vi "Game Controller Teleop.vi"(10 "Match Info":T13={"Autonomous Elapsed Seconds"=0.0, "TeleOp Elapsed Seconds"=0.0, "Disabled Elapsed Seconds"=0.0, "Visited Autonomous"=FALSE, "Visited TeleOp"=FALSE, "Visited Disabled"=FALSE, "Autonomous Settings"={"Autonomous Style"=enum."Independent", "VI Refnum"=refnum}}, 11 "Call Context":T14) -> ()   [LabVIEW 2020]
doc: "This VI is called for each TeleOp packet received from the DS where the robot is not disabled. It is often used to read from the joysticks and update I/O or to update setpoints for timed control loops. It should complete and return within 20 milliseconds or it may miss DS packets."
uses:
  <vilib>/Rock Robotics/WPI/DriverStation/WPI_DriverStationDerivedRobotMode.ctl
  <vilib>/Rock Robotics/WPI/DriverStation/WPI_DriverStationMatch Info.ctl
  Shared Code/TypeDefs/Cluster_Extend HW Outputs.ctl
  Shared Code/TypeDefs/Cluster_FX CloseLoop Values.ctl
  Shared Code/TypeDefs/Cluster_FX Limit Switchs.ctl
  Shared Code/TypeDefs/Cluster_FX Current Values.ctl
  Shared Code/TypeDefs/Cluster_FX Sensor Values.ctl
  Shared Code/TypeDefs/Cluster_FX Integrated Sensor Values.ctl
  Shared Code/TypeDefs/Cluster_Sholder_HW Outputs.ctl
  Shared Code/TypeDefs/Cluster_Wrist HW Outputs.ctl
  Shared Code/TypeDefs/Cluster_Pose Positions.ctl
  Systems/MotionMaser/ENUM_Pose List.ctl
  Type Defs/Cluster_Pigeon Tilt Data.ctl
  Shared Code/TypeDefs/ENUM_Tilt State.ctl
  Systems/SwerveDrive/Cluster_CMD_ACT_Data.ctl
  Shared Code/TypeDefs/ENUM_Swerve_CMD_Mode Select.ctl
  Shared Code/TypeDefs/Cluster_CMD_Direction Data.ctl
  Shared Code/TypeDefs/Cluster_Module Velocity-Direction-Rotations.ctl
  Shared Code/TypeDefs/Level_Velocity plus-minus 1.ctl
  Shared Code/TypeDefs/Dial_Compase heading unit circle CCW positive.ctl
  Type Defs/NUM_Rotate Input.ctl
  Shared Code/TypeDefs/Cluster_X-Y.ctl
  Systems/PigeonIMU/Cluster_CMD_SEN_Data.ctl
  Teleop Support/ENUM_Button Select.ctl
  Teleop Support/ENUM_Axes Select.ctl
  Systems/Extention/Cluster_CMD_ACT_Data.ctl
  Shared Code/TypeDefs/ENUM_Extend_CMD_Mode Select.ctl
  Systems/Sholder/Cluster_CMD_ACT_Data.ctl
  Shared Code/TypeDefs/ENUM_Sholder_CMD_Mode Select.ctl
  Systems/Wrist/Cluster_CMD_ACT_Data.ctl
  Shared Code/TypeDefs/ENUM_Wrist_CMD_Mode Select.ctl
  Systems/Grabber/Cluster_CMD_ACT_Data.ctl
  Shared Code/TypeDefs/ENUM_Grabber_CMD_Mode Select.ctl
  Shared Code/TypeDefs/ENUM_Controller Buzz Select.ctl
  3c76d165-6d6f-4521-944b-83df467126d5.vi
  5b221245-1683-49e4-bbda-b419f5af282c.vi
  8735cd3c-726f-4517-be5d-f0f5cfaf1625.vi
  <vilib>/Rock Robotics/Network Tables/NT Write Boolean.vi
  Systems/Game Controller/Global_SEN_Data Out.vi
  Systems/PigeonIMU/Global_CMD_SEN_Data In.vi
  Systems/Grabber/Global_CMD_ACT_Data In.vi
  Systems/Wrist/Global_CMD_ACT_Data In.vi
  Systems/Extention/Global_ACT_Data Out.vi
  Systems/Sholder/Global_ACT_Data Out.vi
  Systems/Wrist/Global_ACT_Data Out.vi
  Systems/Extention/Global_CMD_ACT_Data In.vi
  Systems/Grabber/Global_ACT_Data Out.vi
  Systems/Game Controller/Global_CMD_Data In.vi
  Systems/SwerveDrive/Global_CMD_ACT_Data In.vi
  Systems/Sholder/Global_CMD_ACT_Data In.vi
  Systems/PigeonIMU/Global_SEN_Data Out.vi
  Systems/SwerveDrive/Global_ACT_Data Out.vi
  <vilib>/Comparison/Equal/Equal Functor/Equal Functor.lvclass
  Systems/Game Controller/GameController_SEN.lvlib
  Systems/SwerveDrive/SwerveDrive_ACT.lvlib
  Systems/PigeonIMU/PigeonIMU_SEN.lvlib
  Systems/Extention/Extend_ACT.lvlib
  Systems/Sholder/Sholder_ACT.lvlib
  Systems/Wrist/Wrist_ACT.lvlib
  Systems/Grabber/Grabber_ACT.lvlib
  Systems/MotionMaser/MotionMaster_SubCMD.lvlib
panel:
  out "Rotation Reduction":dbl
  in  "Balance speed (ft/s)":dbl=10.0
  out "Sen_Pigeon_Tilt Data":T1
  out "Pose":T3
  out "Target  Position Out":T4
  in  "Min Translation Speed (ft/s)":dbl=2.0 format="%#_13g"
  in  "max rotation speed":dbl=0.4
  in  "shoulder speed":dbl=-0.3
  out "ACT_Wrist_HW Output":T5
  out "ACT_Sholder_HW Outputs":T11
  out "ACT_Extend_HW Outputs":T12
  out "POSITION":bool
  in  "funny tilt button":bool
  in  "Drive Deadband":dbl=0.25 format="%#_13g"
  in  "Rotation Deadband":dbl=0.15 format="%#_13g"
  in  "Square Throttle?":bool
  in  "Square Joystick Inputs?":bool
  in  "Max Translation Speed (ft/s)":dbl=16.0 format="%#_13g"
  out "POV":i16
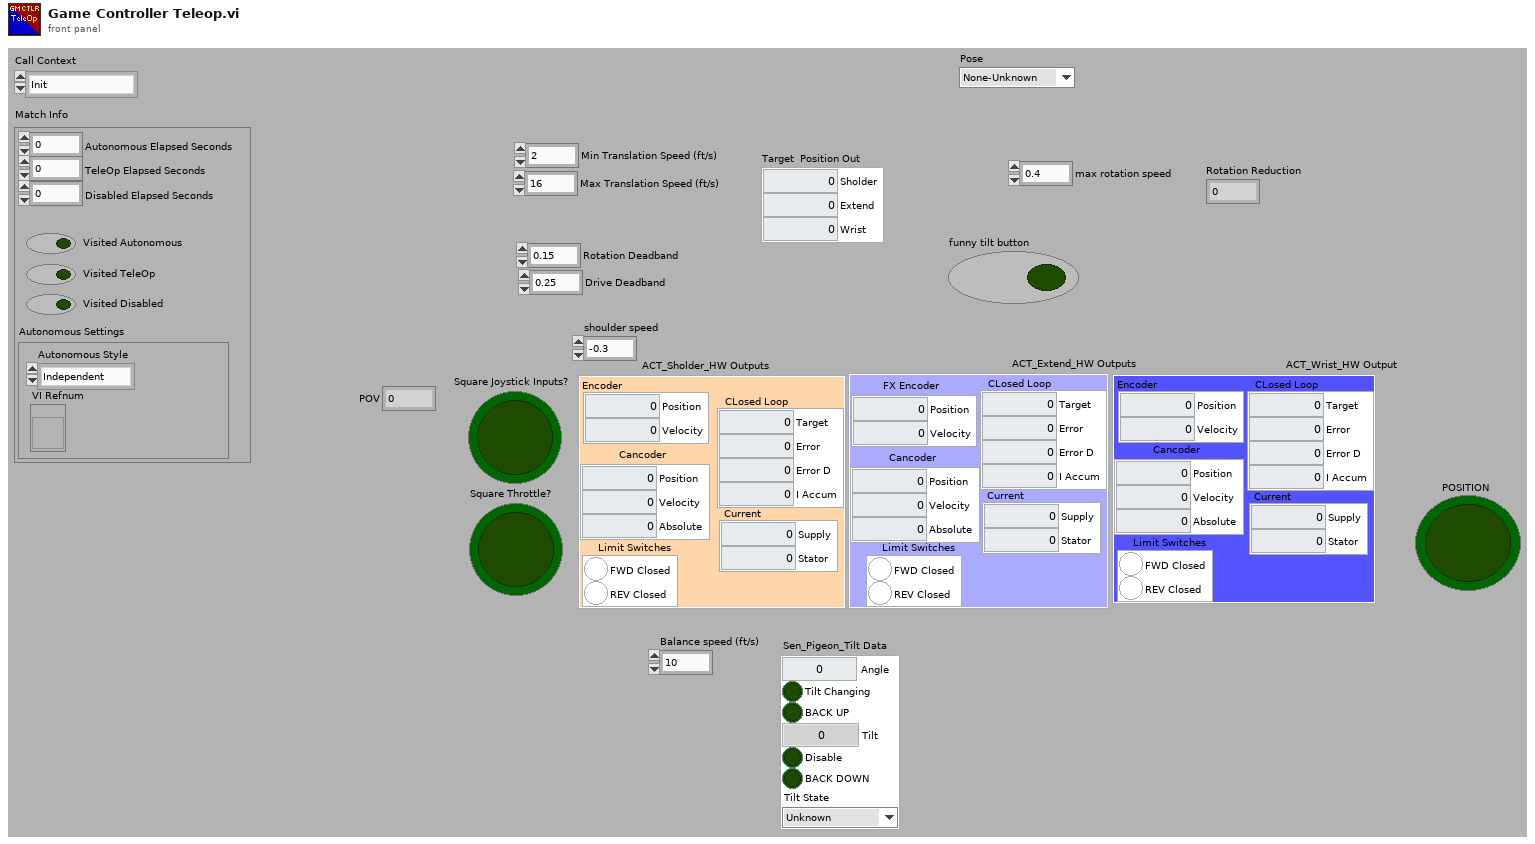
[diagram p1: front panel]
types:
  T1 = typedef "Cluster_Pigeon Tilt Data.ctl" = cluster{"Angle":dbl, "Tilt Changing":bool, "BACK UP":bool, "Tilt":dbl, "Disable":bool, "BACK DOWN":bool, "Tilt State":T2}
  T2 = typedef "ENUM_Tilt State.ctl" = enum16{"Unknown", "Level", "Angle UP from Level", "Level from Angle Up", "Angle Down from Level", "Level from Angle Down"}
  T3 = typedef "MotionMaster_SubCMD.lvlib/ENUM_Pose List.ctl" = enum16{"None-Unknown", "Intake", "Score High", "Score Mid", "Safe Position", "Home Pos"}
  T4 = typedef "Cluster_Pose Positions.ctl" = cluster{"Sholder":i32, "Extend":i32, "Wrist":i32}
  T5 = typedef "Cluster_Wrist HW Outputs.ctl" = cluster{"Encoder":T6, "CLosed Loop":T7, "Limit Switches":T8, "Current":T9, "Cancoder":T10}
  T6 = typedef "Cluster_FX Sensor Values.ctl" = cluster{"Position":i32, "Velocity":i32}
  T7 = typedef "Cluster_FX CloseLoop Values.ctl" = cluster{"Target":dbl, "Error":i32, "Error D":dbl, "I Accum":dbl}
  T8 = typedef "Cluster_FX Limit Switchs.ctl" = cluster{"FWD Closed":bool, "REV Closed":bool}
  T9 = typedef "Cluster_FX Current Values.ctl" = cluster{"Supply":dbl, "Stator":dbl}
  T10 = typedef "Cluster_FX Integrated Sensor Values.ctl" = cluster{"Position":dbl, "Velocity":dbl, "Absolute":dbl}
  T11 = typedef "Cluster_Sholder_HW Outputs.ctl" = cluster{"Encoder":T6, "CLosed Loop":T7, "Limit Switches":T8, "Current":T9, "Cancoder":T10}
  T12 = typedef "Cluster_Extend HW Outputs.ctl" = cluster{"CLosed Loop":T7, "Limit Switches":T8, "Current":T9, "FX Encoder":T6, "Cancoder":T10}
  T13 = typedef "WPI_DriverStationMatch Info.ctl" = cluster{"Autonomous Elapsed Seconds":dbl, "TeleOp Elapsed Seconds":dbl, "Disabled Elapsed Seconds":dbl, "Visited Autonomous":bool, "Visited TeleOp":bool, "Visited Disabled":bool, "Autonomous Settings":cluster{"Autonomous Style":enum16{"Iterative", "Independent"}, "VI Refnum":refnum<vi>}}
  T14 = typedef "WPI_DriverStationDerivedRobotMode.ctl" = enum16{"Init", "Execute", "Stop"}
  T15 = typedef "ENUM_Button Select.ctl" = enum16{"RightPad Green A", "RightPad Red B", "RightPad Blue X", "RightPad Yellow Y", "Left Bump", "Right Bump", "CenterPad Back", "CenterPad Start", "LeftStick Press", "RightStick Press"}
  T16 = typedef "ENUM_Swerve_CMD_Mode Select.ctl" = enum16{"Coast", "Manual", "Auto Trans Auto Rotate", "Manual Trans Auto Rotate", "Balance", "Stop Brake", "Lock Wheels"}
  T17 = typedef "ENUM_Extend_CMD_Mode Select.ctl" = enum16{"STOP", "Position", "Velocity", "Force Home"}
  T18 = typedef "ENUM_Axes Select.ctl" = enum16{"Left Stick Left (-1) Right (1)", "Left Stick Fwd (-1) Back(1)", "Left Trigger (0-1)", "Right Trigger (0-1)", "Right Stick Left(-1 Right (1)", "Right Stick Fwd(-1) Back (1)"}
  T19 = typedef "NUM_Rotate Input.ctl" = dbl
  T20 = typedef "Dial_Compase heading unit circle CCW positive.ctl" = dbl
  T21 = typedef "ENUM_Grabber_CMD_Mode Select.ctl" = enum16{"STOP", "Intake", "Eject"}
  T22 = typedef "Grabber_ACT.lvlib/Cluster_CMD_ACT_Data.ctl" = cluster{"Mode":T21}
  T23 = typedef "Wrist_ACT.lvlib/Cluster_CMD_ACT_Data.ctl" = cluster{"Mode":T24, "Position (counts)":i32, "Velocity (0-1)":dbl}
  T24 = typedef "ENUM_Wrist_CMD_Mode Select.ctl" = enum16{"STOP", "Position", "Speed"}
  T25 = typedef "Sholder_ACT.lvlib/Cluster_CMD_ACT_Data.ctl" = cluster{"Mode":T26, "Position (counts)":i32, "Velocity (0-1)":dbl}
  T26 = typedef "ENUM_Sholder_CMD_Mode Select.ctl" = enum16{"STOP", "Position", "Percent out"}
  T27 = typedef "Extend_ACT.lvlib/Cluster_CMD_ACT_Data.ctl" = cluster{"Mode":T17, "Position (counts)":i32, "Velocity (0-1)":dbl}
  T28 = typedef "PigeonIMU_SEN.lvlib/Cluster_CMD_SEN_Data.ctl" = cluster{"Reset":bool, "Disable":bool}
  T29 = typedef "Cluster_Module Velocity-Direction-Rotations.ctl" = cluster{"Velocity":T30, "Angle":T20, "Rotations Count":dbl}
  T30 = typedef "Level_Velocity plus-minus 1.ctl" = dbl
  T31 = typedef "SwerveDrive_ACT.lvlib/Cluster_CMD_ACT_Data.ctl" = cluster{"Mode":T16, "Direction":T32, "Orientation Robot(t) Field(f)":bool, "Max Translation Speed (ft/sec)":dbl, "Rotation Reduction 1-0":dbl, "Rotation Center From Robot Center":T33, "Auto Angle":T20, "Auto Target (ft)":dbl}
  T32 = typedef "Cluster_CMD_Direction Data.ctl" = cluster{"Traverse":T29, "Rotate(Yaw) CCW 1 CW -1":T19}
  T33 = typedef "Cluster_X-Y.ctl" = cluster{"X":dbl, "Y":dbl}
  T34 = typedef "Cluster_Grabber_SW Outputs.ctl" = cluster{"Enabled":bool, "Closed Loop":bool, "Stalled":bool}
  T35 = typedef "GameController_SEN.lvlib/ENUM_SEN_State.ctl" = enum16{"Startup", "Waiting BUZZ ON", "Shutdown", "Buzzing FULL Timed", "Waiting BUZZ OFF", "Buzzing Cycle Count", "Buzzing Intensity"}
  T36 = typedef "ENUM_Controller Buzz Select.ctl" = enum16{"None", "Timed Full ON", "Set Intensity", ".5 Sec Cycle Count"}
  T37 = typedef "Cluster_Config_Balance Data.ctl" = cluster{"BalancePID Ver":u64, "PID":T38}
  T38 = typedef "Cluster_PID Config.ctl" = cluster{"Gains":T39, "Error Allowed":T40, "I Zone":T40, "Max Out":T41, "Max I Accu":T40, "CL Ramp Rate (S)":dbl}
  T39 = typedef "Cluster_PID Gains.ctl" = cluster{"P":dbl, "I":dbl, "D":dbl, "F":dbl}
  T40 = typedef "Cluster_High-Low.ctl" = cluster{"High":dbl, "Low":dbl}
  T41 = typedef "Cluster_FWD  REV Values.ctl" = cluster{"FWD":dbl, "REV":dbl}
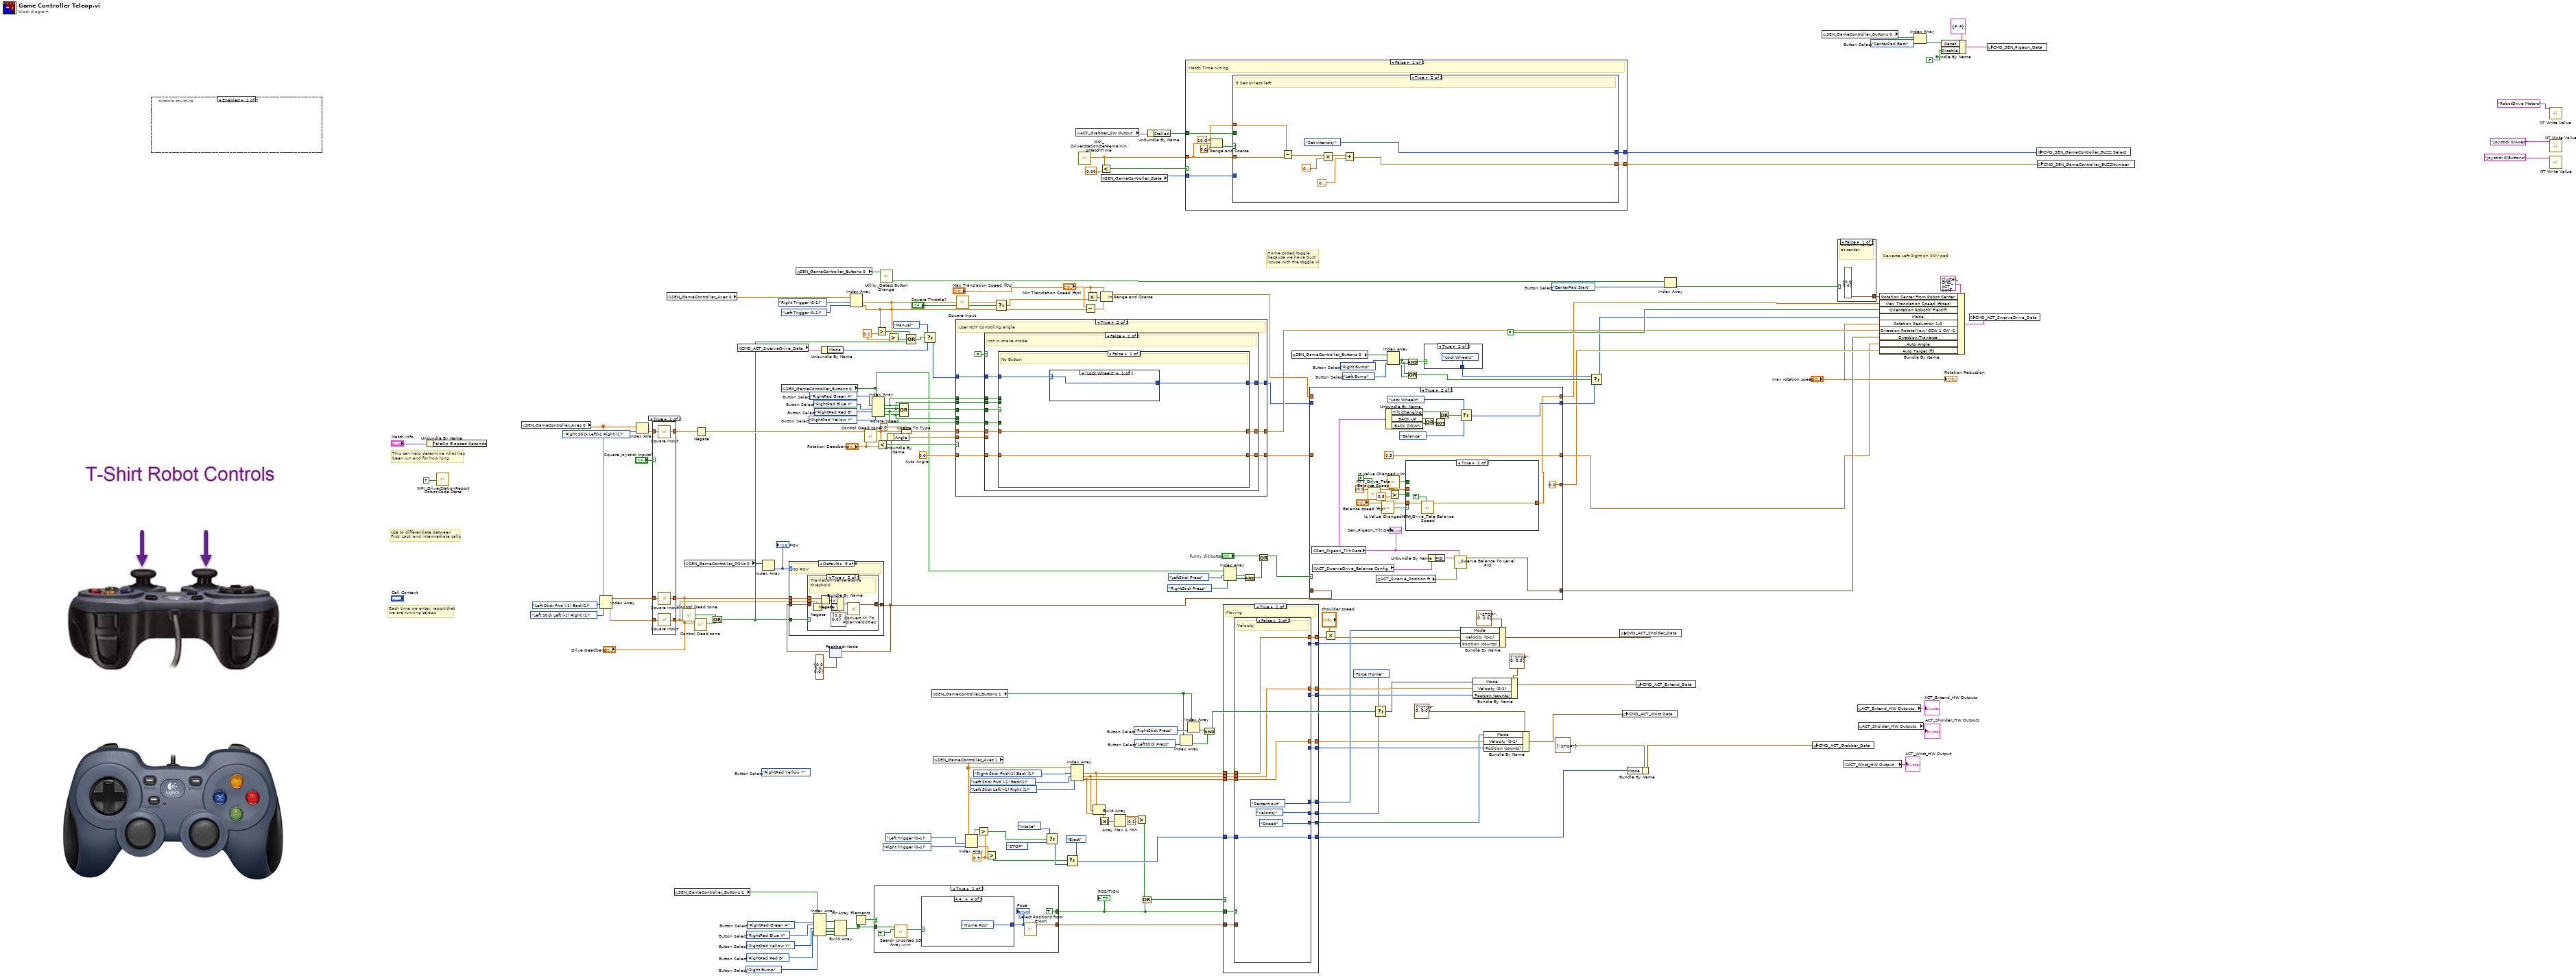
[diagram p0: block diagram]
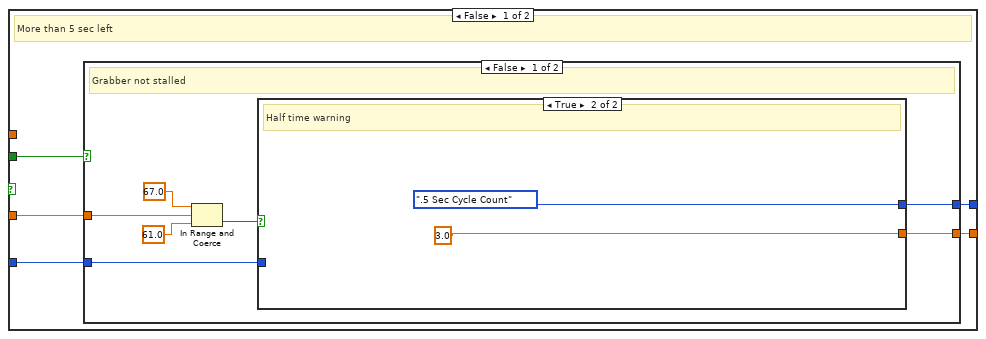
[diagram p2: hidden frame]
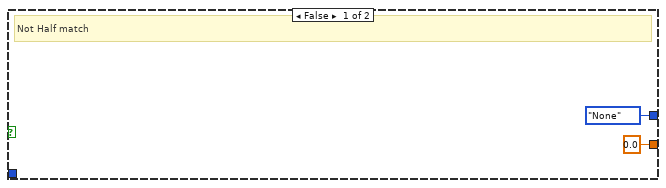
[diagram p3: hidden frame]
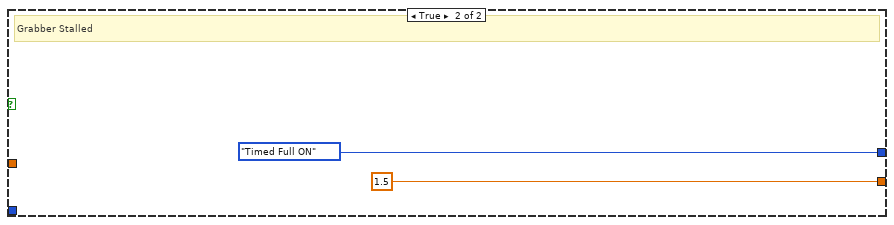
[diagram p4: hidden frame]
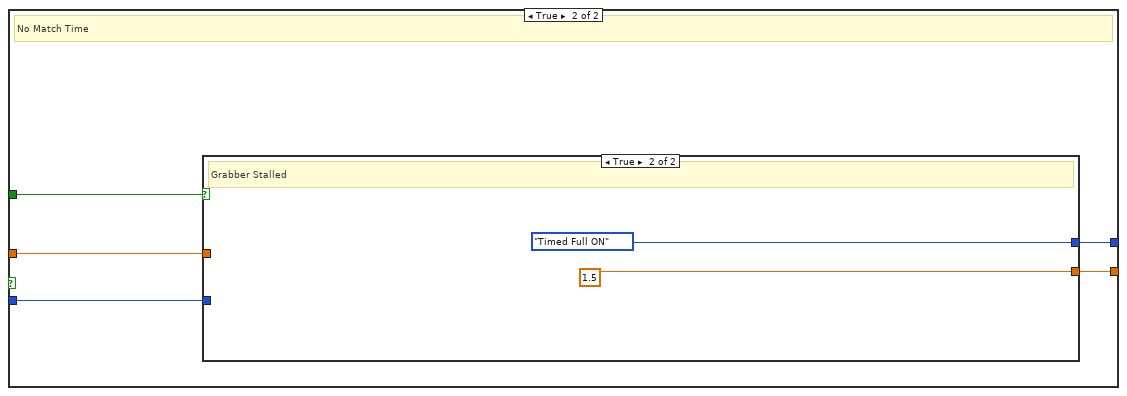
[diagram p5: hidden frame]
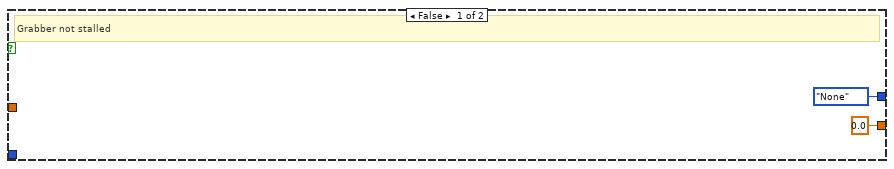
[diagram p6: hidden frame]
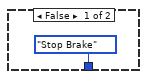
[diagram p7: hidden frame]
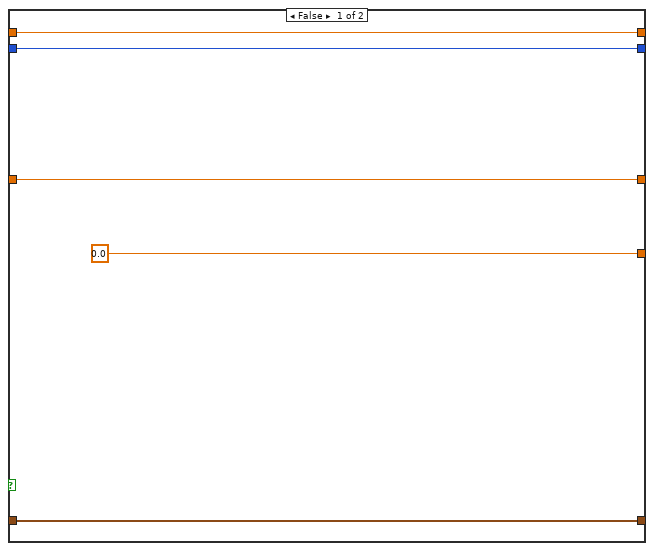
[diagram p8: hidden frame]
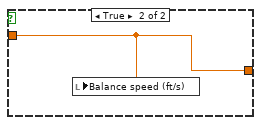
[diagram p11: hidden frame]
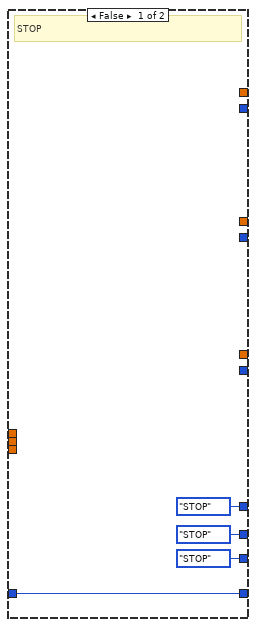
[diagram p12: hidden frame]
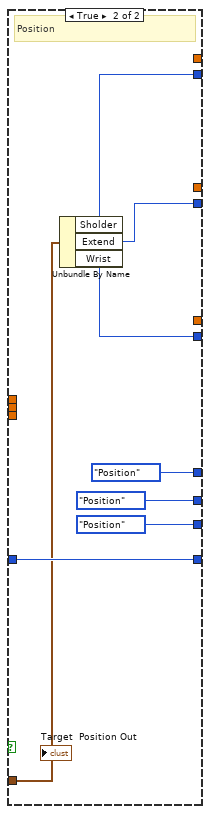
[diagram p13: hidden frame]
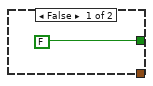
[diagram p14: hidden frame]
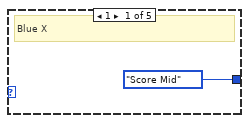
[diagram p15: hidden frame]
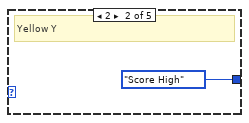
[diagram p16: hidden frame]
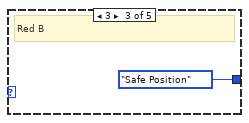
[diagram p17: hidden frame]
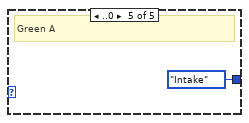
[diagram p18: hidden frame]
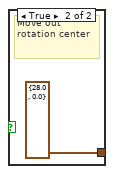
[diagram p19: hidden frame]
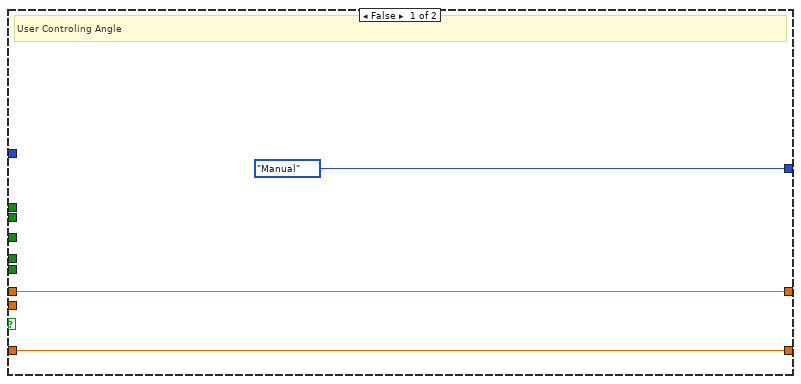
[diagram p20: hidden frame]
diagram:
  w22 = 0.1 ("y")
  w42 = ENUM_Button_Select."Left Bump"  # Button Select
  w51 = ENUM_Button_Select."LeftStick Press"  # Button Select
  w76 = T19 0.0  # Rotate Speed
  w79 = T20 0.0  # Auto Angle
  w82 = ENUM_Button_Select."Right Bump"  # Button Select
  w99 = ENUM_Button_Select."RightPad Red B"  # Button Select
  w100 = ENUM_Button_Select."RightPad Yellow Y"  # Button Select
  w101 = ENUM_Button_Select."RightPad Blue X"  # Button Select
  w102 = ENUM_Button_Select."RightPad Green A"  # Button Select
  (unwired) ENUM_Button_Select."RightPad Yellow Y"  # Button Select
  w109 = 0.9 ("y")
  w145 = ENUM_Button_Select."RightStick Press"  # Button Select
  w155 = ENUM_Button_Select."RightPad Yellow Y"  # Button Select
  w156 = ENUM_Button_Select."RightPad Red B"  # Button Select
  w157 = ENUM_Button_Select."RightPad Blue X"  # Button Select
  w165 = ENUM_Button_Select."CenterPad Start"  # Button Select
  w166 = ENUM_Button_Select."Right Bump"  # Button Select
  w170 = ENUM_Button_Select."CenterPad Back"  # Button Select
  w168 = ENUM_Button_Select."RightPad Green A"  # Button Select
  # "Home coded toggle\nbecause we have trust\nissuse with the toggle VI"
  # "Reverse Left Right on POV pad"
  # "Each time we enter, report that\nwe are running teleop"
  # "Use to differentiate between\nFirst, Last, and Intermediate calls"
  # "This can help determine what has\nbeen run and for how long"
  n1 = disable-structure shown="Enabled" {
    frame Disabled {
      n2 = global read "Global_SEN_Data Out.vi" "SEN_GameController_Axes 1"() -> (w184:dbl[])
      n3 = global read "Global_SEN_Data Out.vi" "SEN_GameController_POVs 1"() -> (w183:i16[])
      n4 = global read "Global_SEN_Data Out.vi" "SEN_GameController_Buttons 1"() -> ()  [unwired: 1 out]
      n5 = Index Array(array=w183) -> ()  [unwired: 1 in, 1 out]
      n6 = Index Array(array=w184) -> ()  [unwired: 1 in, 1 out]
    }
    frame Enabled {
    }
  }
  n7 = Unbundle By Name("Match Info") -> ()  [unwired: 1 out]
  n8 = call <vilib>:"WPI_DriverStationReport Robot Code State.vi"("TeleOp"=TRUE ("Autonomous")) -> ()  [unwired: 10 in, 1 out]
  n9 = global read "Global_SEN_Data Out.vi" "SEN_GameController_Axes 0"() -> (w138:dbl[])
  n10 = Index Array(array=w138, index #1=ENUM_Axes_Select."Left Stick Fwd (-1) Back(1)" ("Axes Select"), index #2=ENUM_Axes_Select."Left Stick Left (-1) Right (1)" ("Axes Select")) -> (element #1=w161:dbl, element #2=w134:dbl)
  n11 = Index Array(array=w138, index=ENUM_Axes_Select."Right Stick Left(-1 Right (1)" ("Axes Select")) -> (element=w136:dbl)
  n12 = case shown="True" "Square Joystick Inputs?" {
    tunnel: [w185 w188] -> w162
    tunnel: [w186 w189] -> w1
    tunnel: [w187 w190] -> w2
    tunnel: w161 -> [w187 w193]
    tunnel: w136 -> [w185 w191]
    tunnel: w134 -> [w186 w192]
    frame False {
    }
    frame True {
      n13 = call "Square Input.vi"("Input"=w191) -> ("Output Squared"=w188:dbl)
      n14 = call "Square Input.vi"("Input"=w193) -> ("Output Squared"=w190:dbl)
      n15 = call "Square Input.vi"("Input"=w192) -> ("Output Squared"=w189:dbl)
    }
  }
  n16 = global read "Global_SEN_Data Out.vi" "SEN_GameController_Axes 0"() -> (w141:dbl[])
  n17 = global read "Global_SEN_Data Out.vi" "SEN_GameController_Buttons 1"() -> (w84:bool[])
  n18 = call "Control Dead zone.vi"("dead zone"="Drive Deadband", "control Value"=w2) -> ("Active"=w69:bool)  [unwired: 8 in, 1 out]
  n19 = global read "Global_SEN_Data Out.vi" "SEN_GameController_POVs 0"() -> (w177:i16[])
  n20 = call "Control Dead zone.vi"("dead zone"="Drive Deadband", "control Value"=w1) -> ("Active"=w70:bool)  [unwired: 8 in, 1 out]
  n21 = Negate(x=w162) -> (-x=w73:dbl)
  n22 = Or(x=w69, y=w70) -> (x .or. y?=w17:bool)
  n23 = global read "Global_CMD_ACT_Data In.vi" "CMD_ACT_SwerveDrive_Data"() -> (w27:T31)
  n24 = Index Array(array=w177) -> (element=w144:i16)  [unwired: 1 in]
  "POV" <- w144
  n25 = global read "Global_SEN_Data Out.vi" "SEN_GameController_Buttons 0"() -> (w16:bool[])
  n26 = global read "Global_SEN_Data Out.vi" "SEN_GameController_Buttons 0"() -> (w53:bool[])
  n27 = Index Array(array=w84, index #1=w102, index #2=w101, index #3=w100, index #4=w99, index #5=w82) -> (element #1=w98:bool, element #2=w97:bool, element #3=w96:bool, element #4=w95:bool, element #5=w81:bool)
  n28 = Unbundle By Name(w27) -> ("Mode"=w20:T16)
  n29 = feedback #1(T29 {"Velocity"=0.0, "Angle"=0.0, "Rotations Count"=0.0} ("Polar Out")) -> (w72:T29)
  n30 = case shown="Default" w144 {
    tunnel: w2 -> [_ _ _ _ _ _ _ _ w230]
    tunnel: w1 -> [_ _ _ _ _ _ _ _ w229]
    tunnel: w72 -> [w197 w201 w205 w209 w213 w217 w221 w225 w228]
    tunnel: [w194 w198 w202 w206 w210 w214 w218 w222 w227] -> w9
    tunnel: w17 -> [_ _ _ _ _ _ _ _ w226]
    frame 0 {
      # "POV Forward"
      n31 = Bundle By Name(cluster=w197, "Velocity"=T30 1.0, "Angle"=T20 0.0) -> (w194:T29)
    }
    frame 45 {
      # "POV Forward Right"
      n32 = Bundle By Name(cluster=w201, "Velocity"=T30 1.0, "Angle"=T20 0.875) -> (w198:T29)
    }
    frame 90 {
      # "POV Right"
      n33 = Bundle By Name(cluster=w205, "Velocity"=T30 1.0, "Angle"=T20 0.75) -> (w202:T29)
    }
    frame 135 {
      # "POV Back Right"
      n34 = Bundle By Name(cluster=w209, "Velocity"=T30 1.0, "Angle"=T20 0.625) -> (w206:T29)
    }
    frame 180 {
      # "POV Back"
      n35 = Bundle By Name(cluster=w213, "Velocity"=T30 1.0, "Angle"=T20 0.5) -> (w210:T29)
    }
    frame 225 {
      # "POV Back Left"
      n36 = Bundle By Name(cluster=w217, "Velocity"=T30 1.0, "Angle"=T20 0.375) -> (w214:T29)
    }
    frame 270 {
      # "POV Left"
      n37 = Bundle By Name(cluster=w221, "Velocity"=T30 1.0, "Angle"=T20 0.25) -> (w218:T29)
    }
    frame 315 {
      # "POV Forward Left"
      n38 = Bundle By Name(cluster=w225, "Velocity"=T30 1.0, "Angle"=T20 0.125) -> (w222:T29)
    }
    frame Default {
      # "NO POV"
      n39 = case shown="True" w226 {
        tunnel: w230 -> [_ w240]
        tunnel: w229 -> [_ w239]
        tunnel: w228 -> [w232 _]
        tunnel: [w233 w236] -> w227
        frame False {
          # "No Translation value"
          n40 = Bundle By Name(cluster=w232, "Velocity"=T30 0.0) -> (w233:T29)
        }
        frame True {
          # "Tranlation Value above threshold"
          n41 = Negate(x=w239) -> (-x=w235:dbl)
          n42 = Negate(x=w240) -> (-x=w234:dbl)
          n43 = Bundle By Name(cluster=T33 {"X"=0.0, "Y"=0.0} ("XY Velocities"), "X"=w234, "Y"=w235) -> (w238:T33)
          n44 = call "Convert XY To Polar Velocities.vi"("XY Velocities"=w238) -> ("Polar Out"=w236:T29)  [unwired: 10 in]
        }
      }
    }
  }
  n45 = feedback-in #1(w9) -> ()
  n46 = Build Array(w98, w97, w96, w95, w81) -> (w93:bool[])
  n47 = Index Array(array=w141, index #1=ENUM_Axes_Select."Right Trigger (0-1)" ("Axes Select"), index #2=ENUM_Axes_Select."Left Trigger (0-1)" ("Axes Select")) -> (element #1=w25:dbl, element #2=w26:dbl)
  n48 = Or Array Elements(Boolean array=w93) -> (logical OR=w94:bool)
  n49 = call "Control Dead zone.vi"("dead zone"="Rotation Deadband", "control Value"=w73) -> ("output Value"=w78:dbl)  [unwired: 8 in, 1 out]
  n50 = Index Array(array=w16, index #1=w168, index #2=w157, index #3=w156, index #4=w155) -> (element #1=w153:bool, element #2=w150:bool, element #3=w152:bool, element #4=w151:bool)
  n51 = case shown="True" w94 {
    tunnel: [_ w243] -> w103
    tunnel: w93 -> [_ w247]
    tunnel: [FALSE TRUE] -> w59
    frame False {
    }
    frame True {
      n52 = call "Search Unsorted 1D Array.vim"("element"=TRUE, "unsorted 1D array"=w247) -> ("index of element"=w245:i32)  [unwired: 9 in]
      n53 = case shown="4.." w245 {
        tunnel: [ENUM_Pose_List."Score Mid" ("Pose") ENUM_Pose_List."Score High" ("Pose") ENUM_Pose_List."Safe Position" ("Pose") ENUM_Pose_List."Home Pos" ("Pose") ENUM_Pose_List."Intake" ("Pose")] -> w242
        frame 1 {
          # "Blue X"
        }
        frame 2 {
          # "Yellow Y"
        }
        frame 3 {
          # "Red B"
        }
        frame 4.. {
        }
        frame ..0 {
          # "Green A"
        }
      }
      "Pose" <- w242
      n54 = call "Select Positions from ENUM.vi"("Pose"=w242) -> ("Selectet  Position Out"=w243:T4)  [unwired: 10 in]
    }
  }
  "POSITION" <- w59
  n55 = Greater?(x=w26, y=w22) -> (0:w23:bool)
  n56 = Less?(x=w78, y="Rotation Deadband") -> (x < y?=w148:bool)
  n57 = call "Utility_Detect Button Change.vi"("HW_Joystick_Buttons"=w53) -> ("Toggle On Rising Out"=w52:bool[])  [unwired: 6 in, 4 out]
  n58 = Greater?(x=w25, y=w22) -> (0:w24:bool)
  n59 = Unbundle By Name(w9) -> ("Angle"=w143:T20)
  n60 = Compound Arithmetic op=OR(w153, w150, w152, w151) -> (w154:bool)
  n61 = Coerce To Type(0:w78, 1:w76) -> (2:w77:T19)
  n62 = Compound Arithmetic op=OR(w23, w24, w17) -> (w21:bool)
  n63 = Select(t=ENUM_Swerve_CMD_Mode_Select."Manual", s=w21, f=w20) -> (s? t:f=w19:T16)
  n64 = global read "Global_SEN_Data Out.vi" "SEN_GameController_Buttons 1"() -> (w50:bool[])
  n65 = global read "Global_SEN_Data Out.vi" "SEN_GameController_Axes 1"() -> (w114:dbl[])
  n66 = case shown="True" w148 {
    tunnel: w77 -> [w253 w267]
    tunnel: w154 -> [_ w266]
    tunnel: w153 -> [_ w265]
    tunnel: w152 -> [_ w264]
    tunnel: w151 -> [_ _]
    tunnel: w150 -> [_ w263]
    tunnel: [w253 w262] -> w80
    tunnel: w143 -> [_ w261]
    tunnel: [ENUM_Swerve_CMD_Mode_Select."Manual" ("Mode") w258] -> w75
    tunnel: w79 -> [w254 w260]
    tunnel: [w254 w259] -> w74
    tunnel: w19 -> [_ w256]
    frame False {
      # "User Controling Angle"
    }
    frame True {
      # "User NOT Controling angle"
      n67 = case shown="False" FALSE {
        tunnel: w267 -> [w269 w301]
        tunnel: w266 -> [w275 w300]
        tunnel: w265 -> [w274 w299]
        tunnel: w264 -> [w273 w298]
        tunnel: w263 -> [w272 w297]
        tunnel: [w269 w296] -> w262
        tunnel: w261 -> [w271 _]
        tunnel: w260 -> [_ w295]
        tunnel: [w270 w294] -> w259
        tunnel: [ENUM_Swerve_CMD_Mode_Select."Manual Trans Auto Rotate" ("Mode") w293] -> w258
        tunnel: w256 -> [_ w292]
        frame True {
          # "in snake mode"
          n68 = case shown="True" w275 {
            tunnel: w274 -> [_ w282]
            tunnel: w273 -> [_ w281]
            tunnel: w272 -> [_ w280]
            tunnel: [w276 w278] -> w270
            tunnel: w271 -> [w276 w277]
            frame False {
              # "No Button"
            }
            frame True {
              # "a,b,x,y Button Pressed"
              n69 = case shown="True" w282 {
                tunnel: w281 -> [w285 _]
                tunnel: [w284 w291] -> w279
                tunnel: w280 -> [w283 _]
                frame False {
                  n70 = case shown="True" w283 {
                    tunnel: w285 -> [w287 _]
                    tunnel: [w286 w290] -> w284
                    frame False {
                      n71 = case shown="False" w287 {
                        tunnel: [w288 w289] -> w286
                        frame False {
                          w288 = T20 0.0  # Auto Angle
                          # "Y"
                        }
                        frame True {
                          w289 = T20 0.25  # Auto Angle
                          # "B"
                        }
                      }
                    }
                    frame True {
                      w290 = T20 0.75  # Auto Angle
                      # "X"
                    }
                  }
                }
                frame True {
                  w291 = T20 0.5  # Auto Angle
                  # "A"
                }
              }
              n72 = Subtract(x=w277, y=w279) -> (x-y=w278:T20)
            }
          }
        }
        frame False {
          # "not in snake mode"
          n73 = case shown="False" w300 {
            tunnel: w301 -> [w305 w309]
            tunnel: w299 -> [_ w314]
            tunnel: w298 -> [_ w313]
            tunnel: w297 -> [_ w312]
            tunnel: [w305 w309] -> w296
            tunnel: w295 -> [w304 w310]
            tunnel: [w304 w311] -> w294
            tunnel: [w303 ENUM_Swerve_CMD_Mode_Select."Manual Trans Auto Rotate" ("Mode")] -> w293
            tunnel: w292 -> [w302 _]
            frame False {
              # "No Button"
              n74 = case shown="\"Lock Wheels\"" w302 {
                selector: w302 -> [w306 _]
                tunnel: [w306 ENUM_Swerve_CMD_Mode_Select."Manual" ("Mode")] -> w303
                frame "Lock Wheels" {
                }
                frame Default {
                }
              }
            }
            frame True {
              # "a,b,x,y Button Pressed"
              n75 = case shown="True" w314 {
                tunnel: w313 -> [w318 _]
                tunnel: [w317 w325] -> w311
                tunnel: w312 -> [w316 _]
                tunnel: w310 -> [w315 _]
                frame False {
                  n76 = case shown="True" w316 {
                    tunnel: w318 -> [w321 _]
                    tunnel: [w320 w324] -> w317
                    tunnel: w315 -> [w319 _]
                    frame False {
                      n77 = case shown="True" w321 {
                        tunnel: [w322 w323] -> w320
                        tunnel: w319 -> [w322 _]
                        frame False {
                          # "Y"
                        }
                        frame True {
                          w323 = T20 0.75  # Auto Angle
                          # "B"
                        }
                      }
                    }
                    frame True {
                      w324 = T20 0.25  # Auto Angle
                      # "X"
                    }
                  }
                }
                frame True {
                  w325 = T20 0.5  # Auto Angle
                  # "A"
                }
              }
            }
          }
        }
      }
    }
  }
  n78 = call "Square Input.vi"("Input"=w25) -> ("Output Squared"=w149:dbl)
  n79 = Index Array(array=w114, index #1=ENUM_Axes_Select."Left Trigger (0-1)" ("Axes Select"), index #2=ENUM_Axes_Select."Right Trigger (0-1)" ("Axes Select")) -> (element #1=w111:dbl, element #2=w110:dbl)
  n80 = Greater?(x=w111, y=w109) -> (0:w108:bool)
  n81 = Greater?(x=w110, y=w109) -> (0:w107:bool)
  n82 = Select(t=w149, s="Square Throttle?", f=w25) -> (s? t:f=w158:dbl)
  n83 = Select(t=ENUM_Grabber_CMD_Mode_Select."Intake" ("Mode"), s=w108, f=ENUM_Grabber_CMD_Mode_Select."STOP" ("Mode")) -> (s? t:f=w115:T21)
  n84 = Select(t=ENUM_Grabber_CMD_Mode_Select."Eject" ("Mode"), s=w107, f=w115) -> (s? t:f=w92:T21)
  n85 = Index Array(array=w114, index #1=ENUM_Axes_Select."Right Stick Fwd(-1) Back (1)" ("Axes Select"), index #2=ENUM_Axes_Select."Left Stick Fwd (-1) Back(1)" ("Axes Select"), index #3=ENUM_Axes_Select."Left Stick Left (-1) Right (1)" ("Axes Select")) -> (element #1=w66:dbl, element #2=w67:dbl, element #3=w68:dbl)
  n86 = global read "Global_ACT_Data Out.vi" "ACT_Grabber_SW Output"() -> (w29:T34)
  n87 = call <vilib>:"WPI_DriverStationGetRemainingMatchTime.vi"() -> ("Match Time(s)"=w31:sgl)  [unwired: 10 in, 1 out]
  n88 = Subtract(x="Min Translation Speed (ft/s)", y=w26) -> (x-y=w55:dbl)
  n89 = Multiply(x="Max Translation Speed (ft/s)", y=w158) -> (x*y=w58:dbl)
  n90 = Build Array(w66, w67, w68) -> (w65:dbl[])
  n91 = Absolute Value(x=w65) -> (abs(x)=w64:dbl[])
  n92 = Less?(x=w31, y=sgl 0.01 ("x")) -> (x < y?=w33:bool)
  n93 = In Range and Coerce(upper limit="Max Translation Speed (ft/s)", x=w58, lower limit=w55) -> (coerced(x)=w57:dbl)  [unwired: 1 out]
  n94 = global read "Global_SEN_Data Out.vi" "SEN_GameController_State"() -> (w32:T35)
  n95 = Array Max & Min(array=w64) -> (max value=w63:dbl)  [unwired: 3 out]
  n96 = Greater?(x=w63, y=0.1) -> (0:w61:bool)
  n97 = Or(x=w61, y=w59) -> (x .or. y?=w60:bool)
  n98 = Unbundle By Name(w29) -> ("Stalled"=w28:bool)
  n99 = Index Array(array=w50, index=w51) -> (element=w48:bool)
  n100 = case shown="False" w33 {
    tunnel: [w331 w364] -> w35
    tunnel: [w330 w361] -> w34
    tunnel: w28 -> [w329 w363]
    tunnel: w31 -> [w328 w362]
    tunnel: w32 -> [w326 w360]
    frame False {
      w327 = sgl 10.0 ("upper limit")
      # "Match Time runing"
      n101 = In Range and Coerce(upper limit=w327, x=w328, lower limit=sgl 0.0) -> (In Range?=w332:bool)  [unwired: 1 out]
      n102 = case shown="True" w332 {
        tunnel: w328 -> [w336 w358]
        tunnel: [w337 ENUM_Controller_Buzz_Select."Set Intensity" ("CMD_SEN_GameController_BUZZ Select")] -> w331
        tunnel: [w335 w352] -> w330
        tunnel: w329 -> [w338 _]
        tunnel: w327 -> [_ w356]
        tunnel: w326 -> [w334 _]
        frame False {
          # "More than 5 sec left"
          n103 = case shown="False" w338 {
            tunnel: [w341 ENUM_Controller_Buzz_Select."Timed Full ON" ("CMD_SEN_GameController_BUZZ Select")] -> w337
            tunnel: w336 -> [w343 _]
            tunnel: [w340 sgl 1.5] -> w335
            tunnel: w334 -> [w339 _]
            frame False {
              # "Grabber not stalled"
              n104 = In Range and Coerce(upper limit=sgl 67.0, x=w343, lower limit=sgl 61.0) -> (In Range?=w342:bool)  [unwired: 1 out]
              n105 = case shown="True" w342 {
                tunnel: [ENUM_Controller_Buzz_Select."None" ("CMD_SEN_GameController_BUZZ Select") ENUM_Controller_Buzz_Select.".5 Sec Cycle Count" ("CMD_SEN_GameController_BUZZ Select")] -> w341
                tunnel: [sgl 0.0 sgl 3.0] -> w340
                tunnel: w339 -> [_ _]
                frame False {
                  # "Not Half match"
                }
                frame True {
                  # "Half time warning"
                }
              }
            }
            frame True {
              # "Grabber Stalled"
            }
          }
        }
        frame True {
          # "5 Sec or less left"
          n106 = Subtract(x=w356, y=w358) -> (x-y=w357:sgl)
          n107 = Multiply(x=w357, y=sgl 0.6) -> (x*y=w355:sgl)
          n108 = Add(x=w355, y=sgl 0.4) -> (x+y=w352:sgl)
        }
      }
    }
    frame True {
      # "No Match Time"
      n109 = case shown="True" w363 {
        tunnel: [ENUM_Controller_Buzz_Select."None" ("CMD_SEN_GameController_BUZZ Select") ENUM_Controller_Buzz_Select."Timed Full ON" ("CMD_SEN_GameController_BUZZ Select")] -> w364
        tunnel: w362 -> [_ _]
        tunnel: [sgl 0.0 sgl 1.5] -> w361
        tunnel: w360 -> [_ _]
        frame False {
          # "Grabber not stalled"
        }
        frame True {
          # "Grabber Stalled"
        }
      }
    }
  }
  n110 = Index Array(array=w50, index=w145) -> (element=w49:bool)
  n111 = And(x=w49, y=w48) -> (x .and. y?=w47:bool)
  n112 = case shown="True" w60 {
    tunnel: [ENUM_Wrist_CMD_Mode_Select."STOP" ("Mode") w388] -> w123
    tunnel: [ENUM_Extend_CMD_Mode_Select."STOP" ("Mode") w387] -> w45
    tunnel: [ENUM_Sholder_CMD_Mode_Select."STOP" ("Mode") w386] -> w122
    tunnel: [w369 w385] -> w119
    tunnel: [_ w383] -> w106
    tunnel: w66 -> [_ w382]
    tunnel: [_ w381] -> w105
    tunnel: w67 -> [_ w380]
    tunnel: w68 -> [_ w379]
    tunnel: [_ w378] -> w104
    tunnel: w103 -> [_ w377]
    tunnel: w92 -> [w369 w384]
    tunnel: [_ w376] -> w88
    tunnel: [_ w375] -> w87
    tunnel: [_ w374] -> w86
    tunnel: w59 -> [_ w373]
    frame False {
      # "STOP"
    }
    frame True {
      # "Moving"
      n113 = case shown="False" w373 {
        tunnel: [ENUM_Wrist_CMD_Mode_Select."Speed" ("Mode") ENUM_Wrist_CMD_Mode_Select."Position" ("Mode")] -> w388
        tunnel: [ENUM_Extend_CMD_Mode_Select."Velocity" ("Mode") ENUM_Extend_CMD_Mode_Select."Position" ("Mode")] -> w387
        tunnel: [ENUM_Sholder_CMD_Mode_Select."Percent out" ("Mode") ENUM_Sholder_CMD_Mode_Select."Position" ("Mode")] -> w386
        tunnel: [w392 w400] -> w385
        tunnel: w384 -> [w392 w400]
        tunnel: [w391 _] -> w383
        tunnel: w382 -> [w391 _]
        tunnel: [w390 _] -> w381
        tunnel: w380 -> [w390 _]
        tunnel: w379 -> [w389 _]
        tunnel: [w389 _] -> w378
        tunnel: w377 -> [_ w399]
        tunnel: [_ w398] -> w376
        tunnel: [_ w397] -> w375
        tunnel: [_ w396] -> w374
        frame False {
          # "Velocity"
        }
        frame True {
          # "Position"
          n114 = Unbundle By Name(w399) -> ("Sholder"=w397:i32, "Extend"=w398:i32, "Wrist"=w396:i32)
          "Target  Position Out" <- w399
        }
      }
    }
  }
  n115 = Index Array(array=w16, index #1=ENUM_Button_Select."LeftStick Press" ("Button Select"), index #2=ENUM_Button_Select."RightStick Press" ("Button Select")) -> (element #1=w12:bool, element #2=w13:bool)
  n116 = And(x=w12, y=w13) -> (x .and. y?=w11:bool)
  n117 = Or(x="funny tilt button", y=w11) -> (x .or. y?=w10:bool)
  n118 = global read "Global_SEN_Data Out.vi" "SEN_GameController_Buttons 0"() -> (w167:bool[])
  n119 = case shown="True" w10 {
    tunnel: w9 -> [w408 _]
    tunnel: [w408 w433] -> w7
    tunnel: w75 -> [w407 _]
    tunnel: [w407 w420] -> w41
    tunnel: w74 -> [w406 _]
    tunnel: [w406 T20 0.5 ("Auto Angle")] -> w3
    tunnel: w57 -> [w405 _]
    tunnel: [w405 w414] -> w6
    tunnel: [0.0 ("Auto Target (ft)") 0.0 ("Auto Target (ft)")] -> w8
    frame False {
    }
    frame True {
      n120 = global read "Global_SEN_Data Out.vi" "Sen_Pigeon_Tilt Data"() -> (w426:T1)
      "Sen_Pigeon_Tilt Data" <- w426
      n121 = global read "Global_ACT_Data Out.vi" "ACT_SwerveDrive_Balance Config"() -> (w432:T37)
      n122 = call "NTV_Drive_Tele Balance Speed.vi"("Read(f) Write(t)"=FALSE, "Balance Speed"=10.0) -> ("Balance Speed"=w410:dbl)  [unwired: 9 in]
      n123 = global read "Global_ACT_Data Out.vi" "ACT_Swerve_Position ft"() -> (w430:dbl)
      n124 = call "Is Value Changed.vim"("value"="Balance speed (ft/s)") -> ("changed or first call?"=w411:bool)
      n125 = Unbundle By Name(w426) -> ("Tilt Changing"=w424:bool, "BACK UP"=w429:bool, "BACK DOWN"=w427:bool)
      n126 = call "Is Value Changed.vim"("value"=w410) -> ("changed or first call?"=w409:bool)
      n127 = Greater?(x=w410, y=0.5) -> (0:w413:bool)
      n128 = case shown="True" w411 {
        tunnel: "Balance speed (ft/s)" -> [w436 w447]
        tunnel: [w435 w445] -> w414
        tunnel: w413 -> [w438 _]
        tunnel: w410 -> [w437 _]
        tunnel: w409 -> [w434 _]
        frame False {
          n129 = case shown="True" w438 {
            tunnel: w437 -> [_ w441]
            tunnel: [w439 w440] -> w435
            tunnel: w436 -> [w439 _]
            tunnel: w434 -> [_ w442]
            frame False {
            }
            frame True {
              n130 = case shown="False" w442 {
                tunnel: w441 -> [w443 w444]
                tunnel: [w443 w444] -> w440
                frame False {
                }
                frame True {
                  n131 = local write "Balance speed (ft/s)"(w444) -> ()
                }
              }
            }
          }
        }
        frame True {
          n132 = call "NTV_Drive_Tele Balance Speed.vi"("Read(f) Write(t)"=TRUE, "Balance Speed"=w447) -> ("Balance Speed"=w445:dbl)  [unwired: 9 in]
        }
      }
      n133 = Or(x=w429, y=w427) -> (x .or. y?=w428:bool)
      n134 = Unbundle By Name(w432) -> ("PID"=w431:T38)
      n135 = Not(x=w428) -> (.not. x?=w425:bool)
      n136 = Or(x=w424, y=w425) -> (x .or. y?=w423:bool)
      n137 = call "Swerve Balance To Level PID.vi"("Yaw Data"=w426, "Position ft"=w430, "Tilt PID Config"=w431) -> ("Output Cluster Out"=w433:T29)  [unwired: 6 in, 2 out]
      n138 = Select(t=ENUM_Swerve_CMD_Mode_Select."Lock Wheels" ("Mode"), s=w423, f=ENUM_Swerve_CMD_Mode_Select."Balance" ("Mode")) -> (s? t:f=w420:T16)
    }
  }
  n139 = Multiply(x="shoulder speed", y=w106) -> (x*y=w85:dbl)
  n140 = Select(t=ENUM_Extend_CMD_Mode_Select."Force Home" ("Mode"), s=w47, f=w45) -> (s? t:f=w44:T17)
  n141 = Index Array(array=w167, index #1=w166, index #2=w42) -> (element #1=w38:bool, element #2=w39:bool)
  n142 = Or(x=w39, y=w38) -> (x .or. y?=w37:bool)
  n143 = And(x=w38, y=w39) -> (x .and. y?=w36:bool)
  n144 = case shown="True" w36 {
    tunnel: [ENUM_Swerve_CMD_Mode_Select."Stop Brake" ("t") ENUM_Swerve_CMD_Mode_Select."Lock Wheels" ("t")] -> w40
    frame False {
    }
    frame True {
    }
  }
  n145 = Bundle By Name(cluster=T25 {"Mode"=enum."STOP", "Position (counts)"=0, "Velocity (0-1)"=0.0} ("CMD_ACT_Template_Data"), "Mode"=w122, "Velocity (0-1)"=w85, "Position (counts)"=w87) -> (w129:T25)
  n146 = Bundle By Name(cluster=T27 {"Mode"=enum."STOP", "Position (counts)"=0, "Velocity (0-1)"=0.0} ("CMD_ACT_Template_Data"), "Mode"=w44, "Velocity (0-1)"=w105, "Position (counts)"=w88) -> (w131:T27)
  n147 = Bundle By Name(cluster=T23 {"Mode"=enum."STOP", "Position (counts)"=0, "Velocity (0-1)"=0.0} ("CMD_ACT_Template_Data"), "Mode"=w123, "Velocity (0-1)"=w104, "Position (counts)"=w86) -> (w127:T23)
  n148 = Select(t=w40, s=w37, f=w41) -> (s? t:f=w5:T16)
  n149 = global write "Global_CMD_ACT_Data In.vi" "CMD_ACT_Sholder_Data"(w129) -> ()
  n150 = global write "Global_CMD_ACT_Data In.vi" "CMD_ACT_Wrist Data"(w127) -> ()
  n151 = Bundle By Name(cluster=T22 {"Mode"=enum."STOP"} ("CMD_Wrist_Template_Data"), "Mode"=w119) -> (w120:T22)
  n152 = global write "Global_CMD_ACT_Data In.vi" "CMD_ACT_Extend_Data"(w131) -> ()
  n153 = Index Array(array=w52, index=w165) -> (element=w164:bool)
  n154 = global write "Global_CMD_ACT_Data In.vi" "CMD_ACT_Grabber_Data"(w120) -> ()
  n155 = global read "Global_SEN_Data Out.vi" "SEN_GameController_Buttons 0"() -> (w140:bool[])
  n156 = case shown="False" w164 {
    tunnel: [T33 {"X"=0.0, "Y"=0.0} ("Rotation Center From Robot Center") T33 {"X"=28.0, "Y"=0.0} ("Rotation Center From Robot Center")] -> w163
    frame False {
      # "Rotation center at center"
    }
    frame True {
      # "Move out rotation center"
    }
  }
  n157 = global read "Global_ACT_Data Out.vi" "ACT_Wrist_HW Output"() -> (→"ACT_Wrist_HW Output":T5)
  n158 = global read "Global_ACT_Data Out.vi" "ACT_Extend_HW Outputs"() -> (→"ACT_Extend_HW Outputs":T12)
  n159 = global read "Global_ACT_Data Out.vi" "ACT_Sholder_HW Outputs"() -> (→"ACT_Sholder_HW Outputs":T11)
  n160 = Bundle By Name(cluster=T31 {"Mode"=enum."Coast", "Direction"={"Traverse"={"Velocity"=0.0, "Angle"=0.0, "Rotations Count"=0.0}, "Rotate(Yaw) CCW 1 CW -1"=0.0}, "Orientation Robot(t) Field(f)"=FALSE, "Max Translation Speed (ft/sec)"=0.0, "Rotation Reduction 1-0"=0.0, "Rotation Center From Robot Center"={"X"=0.0, "Y"=0.0}, "Auto Angle"=0.0, "Auto Target (ft)"=0.0} ("CMD_ACT_Template_Data"), "Rotation Center From Robot Center"=w163, "Max Translation Speed (ft/sec)"=w6, "Orientation Robot(t) Field(f)"=FALSE, "Mode"=w5, "Rotation Reduction 1-0"="max rotation speed", "Direction.Rotate(Yaw) CCW 1 CW -1"=w80, "Direction.Traverse"=w7, "Auto Angle"=w3, "Auto Target (ft)"=w8) -> (w175:T31)
  n161 = Index Array(array=w140, index=w170) -> (element=w171:bool)
  n162 = Bundle By Name(cluster=T28 {"Reset"=FALSE, "Disable"=FALSE} ("CMD_SEN_Pigeon_Data"), "Reset"=w171, "Disable"=FALSE) -> (w172:T28)
  n163 = global write "Global_CMD_ACT_Data In.vi" "CMD_ACT_SwerveDrive_Data"(w175) -> ()
  n164 = global write "Global_CMD_SEN_Data In.vi" "CMD_SEN_Pigeon_Data"(w172) -> ()
  n165 = global write "Global_CMD_Data In.vi" "CMD_SEN_GameController_BUZZ Select"(w35) -> ()
  n166 = global write "Global_CMD_Data In.vi" "CMD_SEN_GameController_BUZZNumber"(w34) -> ()
  n167 = call-poly <vilib>:"NT Write Value.vi"("name"="RobotDrive Motors" ("Name")) -> ()  [unwired: 10 in, 1 out]
  n168 = call-poly <vilib>:"NT Write Value.vi"("name"="Joystick 0/Axes" ("Name")) -> ()  [unwired: 10 in, 1 out]
  n169 = call-poly <vilib>:"NT Write Value.vi"("name"="Joystick 0/Buttons" ("Name")) -> ()  [unwired: 10 in, 1 out]
  "Rotation Reduction" <- "max rotation speed"
